vi "Replace HDI.vi"(8 "error in":errorcluster, 9 "Slot":i32, 10 "Chuck":i32, 11 "PickerTool in":refnum<class "PickerTool Class.lvclass">) -> (0 "error out":errorcluster, 3 "PickerTool out":refnum<class "PickerTool Class.lvclass">)   [LabVIEW 2011, in "PickerTool Class.lvclass"]
uses:
  PickerTool Class.lvclass
  Config Manager Class/Type Definitions/Part Type.ctl
  Config Manager Class/Type Definitions/Offset.ctl
  WorkTable Class/WorkTable Class.lvclass
  Vec3d Class/Vec3d Class.lvclass
  Config Manager Class/Config Manager Class.lvclass
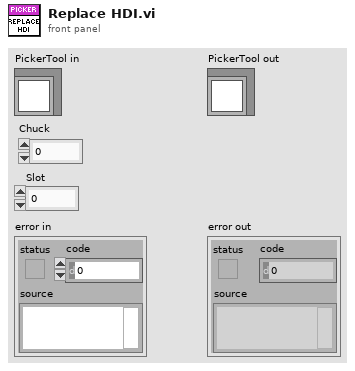
[diagram p1: front panel]
types:
  T1 = enum16{"Empty", "Bare HDI", "Unglued", "Stamped", "PartOnTop", "Weighted", "Unpotted", "Potted"}
  T2 = typedef "Part Type.ctl" = enum16{"BBM", "HDI", "BARE HDI", "GLUERESERVOIR", "STAMP_1", "STAMP_2", "STAMP_3", "STAMP_4", "STAMP_5", "WEIGHT_1", "WEIGHT_2", "WEIGHT_3", "WEIGHT_4", "WEIGHT_5", "WEIGHT_6", "WEIGHT_7", "WEIGHT_8", "PICKER_TOOL", "GRABER_TOOL"}
  T3 = typedef "Offset.ctl" = enum16{"needle_offset", "tool_holder_offset"}
  T4 = typedef "Worktable_Module Slot.ctl" = cluster{"Slot State":enum16{"Empty", "Bare HDI", "Unglued", "Stamped", "PartOnTop", "Weighted", "Unpotted", "Potted"}, "BBM Type":enum16{"None", "BBM", "GlassSlide"}, "HDI Type":enum16{"None", "HDI", "Polyimide"}, "Vacuum Channel":u8, "Location/Orientation BBM":T5, "Location/Orientation HDI":T5, "S/N":string}
  T5 = typedef "Position_Orientation.ctl" = cluster{"Center":refnum<class "Vec3d Class.lvclass">, "Orientation":refnum<class "Orient3d Class.lvclass">}
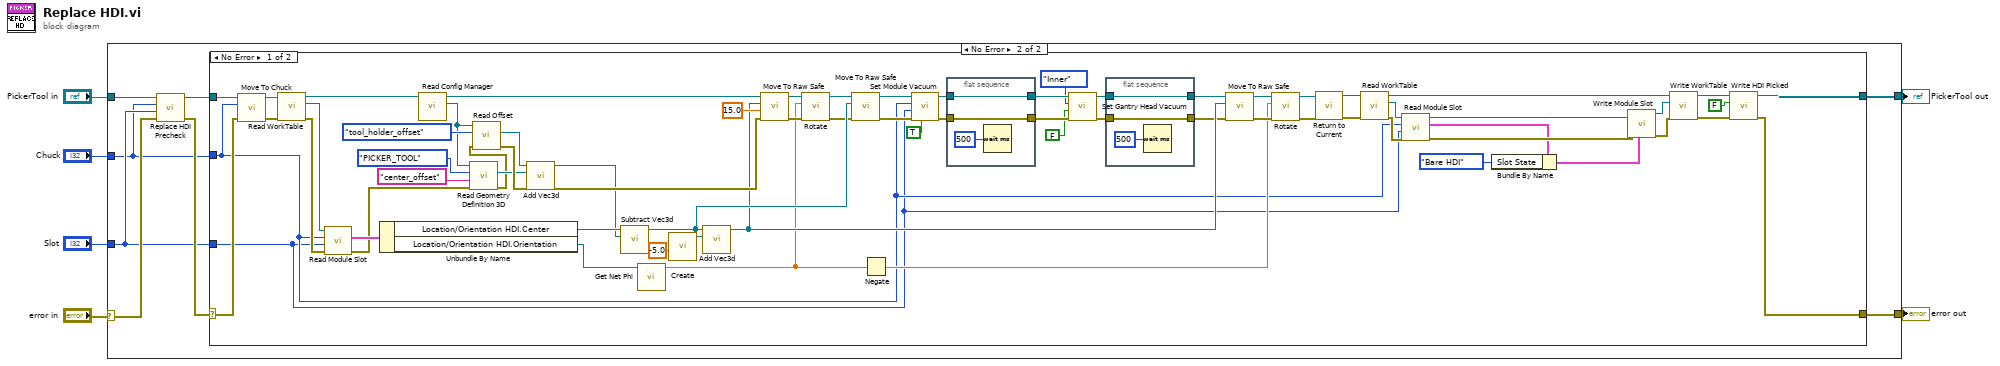
[diagram p0: block diagram]
diagram:
  n1 = case shown="No Error" "error in" {
    selector: "error in" -> [w7 w15]
    tunnel: [w7 w14] -> w5
    tunnel: [w8 w13] -> w3
    tunnel: "PickerTool in" -> [w8 w16]
    tunnel: "Slot" -> [_ w10]
    tunnel: "Chuck" -> [_ w9]
    frame Error {
    }
    frame No Error {
      n2 = call "Replace HDI Precheck.vi"("error in"=w15, "Slot Number in"=w10, "Chuck Number in"=w9, "PickupTool Class in"=w16) -> ("error out"=w11:errorcluster, "PickupTool Class out"=w12:refnum<class "PickerTool Class.lvclass">)  [unwired: 6 in]
      n3 = case shown="No Error" w11 {
        selector: w11 -> [w84 w93]
        tunnel: [w19 w93] -> w14
        tunnel: w12 -> [w85 w92]
        tunnel: [w18 w92] -> w13
        tunnel: w10 -> [w23 _]
        tunnel: w9 -> [w24 _]
        frame No Error {
          n4 = call-dynamic "Move To Chuck.vi"("error in"=w84, "Chuck"=w24, "Gantry in"=w85) -> ("error out"=w73:errorcluster, "Gantry out"=w77:refnum<class "PickerTool Class.lvclass">)  [unwired: 7 in]
          n5 = call-dynamic "Read WorkTable.vi"("error in"=w73, "Gantry Class in"=w77) -> ("error out"=w82:errorcluster, "WorkTable Class.lvclass"=w83:refnum<class "WorkTable Class.lvclass">, "Gantry Class out"=w76:refnum<class "PickerTool Class.lvclass">)  [unwired: 7 in]
          n6 = call-dynamic "Read Module Slot.vi"("error in"=w82, "slot"=w23, "chuck"=w24, "WorkTable in"=w83) -> ("error out"=w39:errorcluster, "Module Slot"=w81:T4)  [unwired: 5 in, 1 out]
          n7 = Unbundle By Name(w81) -> ("Location/Orientation HDI.Center"=w71:refnum<class "Vec3d Class.lvclass">, "Location/Orientation HDI.Orientation"=w65:refnum<class "Orient3d Class.lvclass">)
          n8 = call-dynamic "Read Config Manager.vi"("Gantry in"=w76) -> ("Config Manager"=w41:refnum<class "Config Manager Class.lvclass">, "Gantry out"=w75:refnum<class "PickerTool Class.lvclass">)  [unwired: 8 in, 1 out]
          n9 = call "Read Geometry Definition 3D.vi"("error in"=w39, "Feature"="center_offset", "Part Type"=Part_Type."PICKER_TOOL", "Config Manager in"=w41) -> ("error out"=w40:errorcluster, "Feature Coordinates"=w42:refnum<class "Vec3d Class.lvclass">)  [unwired: 5 in, 1 out]
          n10 = call "Read Offset.vi"("error in"=w40, "Offset"=Offset."tool_holder_offset", "Config Manager in"=w41) -> ("error out"=w72:errorcluster, "Vec3d out"=w80:refnum<class "Vec3d Class.lvclass">)  [unwired: 6 in, 1 out]
          n11 = call-dynamic "Add Vec3d.vi"("error in (no error)"=w72, 10:"Vec3d Class in"=w42, 11:"Vec3d Class in"=w80) -> ("error out"=w78:errorcluster, "Vec3d Class out"=w70:refnum<class "Vec3d Class.lvclass">)  [unwired: 7 in]
          n12 = call "Subtract Vec3d.vi"("Vec3d in 2"=w70, "Vec3d in 1"=w71) -> ("Vec3d Class out"=w67:refnum<class "Vec3d Class.lvclass">)  [unwired: 8 in, 1 out]
          n13 = call "Get Net Phi.vi"("Orient3d"=w65) -> ("phi(deg)"=w36:dbl)  [unwired: 8 in, 2 out]
          n14 = call "Create.vi"("Z"=-5.0) -> ("Vec3d Class out"=w68:refnum<class "Vec3d Class.lvclass">)  [unwired: 9 in, 1 out]
          n15 = call-dynamic "Add Vec3d.vi"(10:"Vec3d Class in"=w68, 11:"Vec3d Class in"=w67) -> ("Vec3d Class out"=w66:refnum<class "Vec3d Class.lvclass">)  [unwired: 8 in, 1 out]
          n16 = call-dynamic "Move To Raw Safe.vi"("error in"=w78, "Speed(mm/s)"=15.0 ("Speed"), "Destination"=w66, "Gantry in"=w75) -> ("error out"=w62:errorcluster, "Gantry out"=w64:refnum<class "PickerTool Class.lvclass">)  [unwired: 6 in]
          n17 = call-dynamic "Rotate.vi"("error in"=w62, "distance(deg)"=w36, "Gantry in"=w64) -> ("error out"=w61:errorcluster, "Gantry out"=w63:refnum<class "PickerTool Class.lvclass">)  [unwired: 7 in]
          n18 = call-dynamic "Move To Raw Safe.vi"("error in"=w61, "Destination"=w67, "Gantry in"=w63) -> ("error out"=w50:errorcluster, "Gantry out"=w52:refnum<class "PickerTool Class.lvclass">)  [unwired: 7 in]
          n19 = Negate(x=w36) -> (-x=w56:dbl)
          n20 = call-dynamic "Set Module Vacuum.vi"("On/Off"=TRUE, "error in"=w50, "Slot Number"=w23, "Chuck Number"=w24, "Gantry in"=w52) -> ("error out"=w43:errorcluster, "Gantry out"=w53:refnum<class "PickerTool Class.lvclass">)  [unwired: 5 in]
          n21 = flat-sequence {
            tunnel: w53 -> [w88]
            tunnel: [w88] -> w49
            tunnel: w43 -> [w87]
            tunnel: [w87] -> w46
            frame #0 {
              n22 = Wait (ms)(milliseconds to wait=u32 500) -> ()  [unwired: 1 out]
            }
          }
          n23 = call-dynamic "Set Gantry Head Vacuum.vi"("error in (no error)"=w46, "On/Off"=FALSE, "Inner/Outer"=enum16{"Outer", "Inner"}."Inner", "Gantry Class in"=w49) -> ("error out"=w47:errorcluster, "Gantry Class out"=w48:refnum<class "PickerTool Class.lvclass">)  [unwired: 6 in]
          n24 = flat-sequence {
            tunnel: w48 -> [w91]
            tunnel: [w91] -> w55
            tunnel: w47 -> [w90]
            tunnel: [w90] -> w54
            frame #0 {
              n25 = Wait (ms)(milliseconds to wait=u32 500) -> ()  [unwired: 1 out]
            }
          }
          n26 = call-dynamic "Move To Raw Safe.vi"("error in"=w54, "Destination"=w66, "Gantry in"=w55) -> ("error out"=w58:errorcluster, "Gantry out"=w60:refnum<class "PickerTool Class.lvclass">)  [unwired: 7 in]
          n27 = call-dynamic "Rotate.vi"("error in"=w58, "distance(deg)"=w56, "Gantry in"=w60) -> ("error out"=w57:errorcluster, "Gantry out"=w59:refnum<class "PickerTool Class.lvclass">)  [unwired: 7 in]
          n28 = call-dynamic "Return to Current.vi"("error in"=w57, "Gantry in"=w59) -> ("error out"=w25:errorcluster, "Gantry out"=w26:refnum<class "PickerTool Class.lvclass">)  [unwired: 8 in]
          n29 = call-dynamic "Read WorkTable.vi"("error in"=w25, "Gantry Class in"=w26) -> ("error out"=w30:errorcluster, "WorkTable Class.lvclass"=w35:refnum<class "WorkTable Class.lvclass">, "Gantry Class out"=w34:refnum<class "PickerTool Class.lvclass">)  [unwired: 7 in]
          n30 = call-dynamic "Read Module Slot.vi"("error in"=w30, "slot"=w23, "chuck"=w24, "WorkTable in"=w35) -> ("error out"=w31:errorcluster, "Module Slot"=w28:T4, "WorkTable out"=w29:refnum<class "WorkTable Class.lvclass">)  [unwired: 5 in]
          n31 = Bundle By Name(cluster=w28, "Slot State"=T1."Bare HDI") -> (w27:T4)
          n32 = call-dynamic "Write Module Slot.vi"("Module Slot"=w27, "error in"=w31, "WorkTable in"=w29) -> ("error out"=w32:errorcluster, "WorkTable out"=w33:refnum<class "WorkTable Class.lvclass">)  [unwired: 7 in]
          n33 = call-dynamic "Write WorkTable.vi"("error in (no error)"=w32, "WorkTable Class.lvclass"=w33, "Gantry Class in"=w34) -> ("error out"=w20:errorcluster, "Gantry Class out"=w21:refnum<class "PickerTool Class.lvclass">)  [unwired: 7 in]
          n34 = call "Write HDI Picked.vi"("error in (no error)"=w20, "HDI Picked"=FALSE, "PickerTool Class in"=w21) -> ("error out"=w19:errorcluster, "PickerTool Class out"=w18:refnum<class "PickerTool Class.lvclass">)  [unwired: 7 in]
        }
        frame Error {
        }
      }
    }
  }
  "error out" <- w5
  "PickerTool out" <- w3
